vi "setLaserPower.vi"(1 "laser power (mW)":dbl, 2 "laser":T1) -> (0 "laser power changed":bool)   [LabVIEW 2015]
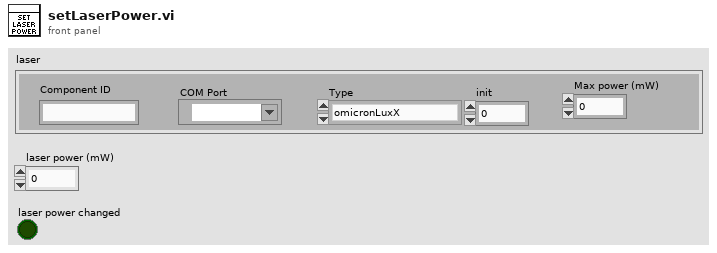
[diagram p1: front panel]
types:
  T1 = cluster{"Component ID":string, "COM Port":refnum<visa-resource-name>, "Type ":enum16{"omicronLuxX", "coherentObis"}, "init":i16, "Max power (mW)":dbl}
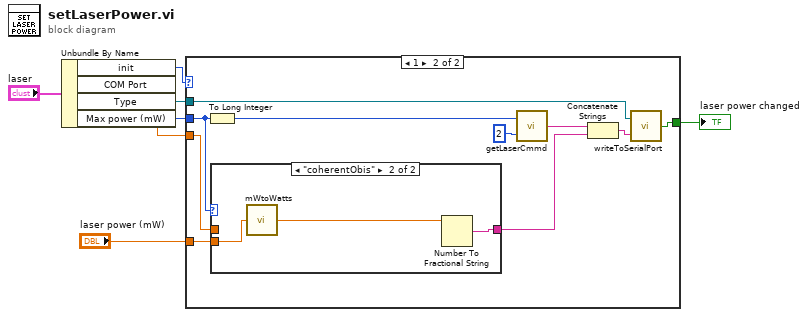
[diagram p0: block diagram]
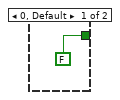
[diagram p2: hidden frame]
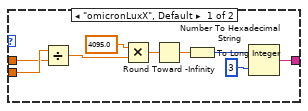
[diagram p3: hidden frame]
diagram:
  n1 = Unbundle By Name("laser") -> ("init"=w5:i16, "COM Port"=w6:refnum<visa-resource-name>, "Type"=w7:enum16{"omicronLuxX", "coherentObis"}, "Max power (mW)"=w1:dbl)
  n2 = case shown="1" w5 {
    tunnel: w6 -> [_ w11]
    tunnel: w7 -> [_ w16]
    tunnel: [FALSE ("data written to port?") w12] -> w4
    tunnel: "laser power (mW)" -> [_ w15]
    tunnel: w1 -> [_ w9]
    frame 0, Default {
    }
    frame 1 {
      n3 = To Long Integer(number=w16) -> (32bit integer=w17:i32)
      n4 = case shown="\"coherentObis\"" w16 {
        tunnel: w15 -> [w27 w30]
        tunnel: [w19 w28] -> w13
        tunnel: w9 -> [w26 _]
        frame "omicronLuxX", Default {
          n5 = Divide(x=w27, y=w26) -> (x/y=w24:dbl)
          n6 = Multiply(x=4095.0 ("number"), y=w24) -> (x*y=w20:dbl)
          n7 = Round Toward -Infinity(1:w20) -> (0:w22:dbl)
          n8 = To Long Integer(number=w22) -> (32bit integer=w23:i32)
          n9 = Number To Hexadecimal String(1:i16 3 ("width (-)"), 2:w23) -> (0:w19:string)
        }
        frame "coherentObis" {
          n10 = call "mWtoWatts.vi"("mW"=w30) -> ("W"=w29:dbl)
          n11 = Number To Fractional String(number=w29) -> (F-format string=w28:string)  [unwired: 3 in]
        }
      }
      n12 = call "getLaserCmmd.vi"("Cmmd index"=2, "Laser type"=w17) -> ("Laser command"=w14:string)
      n13 = Concatenate Strings(w14, w13) -> (w10:string)
      n14 = call "writeToSerialPort.vi"("Cmmd"=w10, "input COM Port"=w11) -> ("data written to port?"=w12:bool)
    }
  }
  "laser power changed" <- w4
